vi "mks946_record_SC.vi"(9 "value_array":dbl[](array[numeric]), 11 "time":timestamp) -> (0 "status":bool)   [LabVIEW 2019]
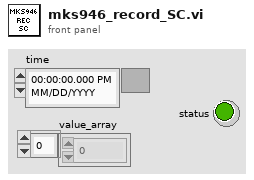
[diagram p1: front panel]
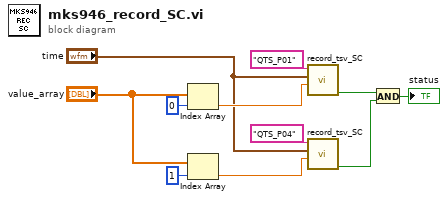
[diagram p0: block diagram]
diagram:
  n1 = Index Array(array="value_array", index=0) -> (element=w7:dbl)
  n2 = Index Array(array="value_array", index=1) -> (element=w6:dbl)
  n3 = call "record_tsv_SC.vi"("value"=w7, "time"="time", "var_name"="QTS_P01") -> ("status"=w3:bool)  [unwired: 7 in, 1 out]
  n4 = call "record_tsv_SC.vi"("value"=w6, "time"="time", "var_name"="QTS_P04") -> ("status"=w1:bool)  [unwired: 7 in, 1 out]
  n5 = And(x=w3, y=w1) -> (x .and. y?=→"status":bool)
